vi "VariaveisMedicao.vi"() -> ()   [LabVIEW 2019]
panel:
  in  "MemoriasSetInfoInversor":T1(array[cluster])
  in  "CorrenteAero":cluster{"X":dbl, "Y":dbl}[](array[cluster])
  in  "TensaoAero":cluster{"X":dbl, "Y":dbl}[](array[cluster])
  in  "Anemometro2":cluster{"X":dbl, "Y":dbl}[](array[cluster])
  in  "Anemometro1":cluster{"X":dbl, "Y":dbl}[](array[cluster])
  in  "VelocidadeExaustor":cluster{"X":dbl, "Y":dbl}[](array[cluster])
  in  "OndaCont":cluster{"X":dbl, "Y":dbl}[](array[cluster])
  in  "GraphSenoide":cluster{"X":dbl, "Y":dbl}[](array[cluster])
  in  "GraphPontos":cluster{"X":dbl, "Y":dbl}[](array[cluster])
  out "MemoriasPlayInversor":T2(array[cluster])
  out "MemoriasStatusInversor":T3(array[cluster])
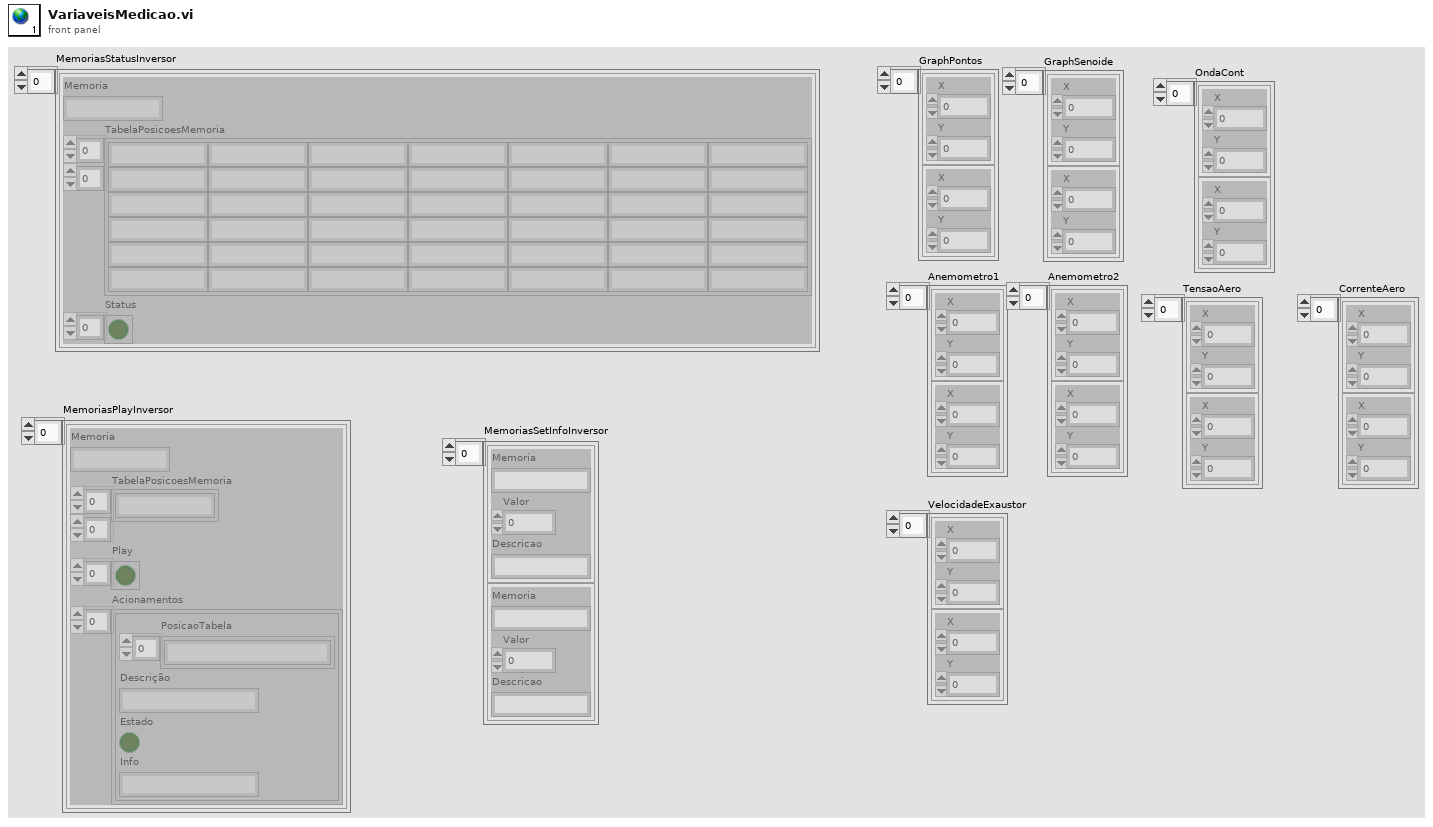
[diagram p1: front panel]
types:
  T1 = cluster{"Memoria":string, "Valor":i16, "Descricao":string}[]
  T2 = cluster{"Memoria":string, "TabelaPosicoesMemoria":string[][], "Play":bool[], "Acionamentos":cluster{"PosicaoTabela":string[], "Descrição":string, "Estado":bool, "Info":string}[]}[]
  T3 = cluster{"Memoria":string, "TabelaPosicoesMemoria":string[][], "Status":bool[]}[]
diagram:
